vi "GetIntegrationMetaData.vi"(8 "error in":errorcluster, 11 "Datawarehouse in":refnum<class "Datawarehouse.lvclass">) -> (0 "error out":errorcluster, 2 "IntegrationMetaData":string, 3 "Datawarehouse out":refnum<class "Datawarehouse.lvclass">)   [LabVIEW 2021, in "ProligentXMLGenerator.lvlib" / "Datawarehouse.lvclass"]
doc: "The information contained in this attribute is saved in the data warehouse as is. It can\nbe used by the integrator to add some meta data that will help him later to troubleshoot his\nintegration. This meta data is stored in the F_INTEGRATION_METADATA column of the T_FACT_DELIVERY_SOURCE\ntable.\n\nThis value is limited to 2000 charactesrs and must no be empty."
uses:
  Datawarehouse.lvclass
  Datawarehouse.lvclass/Datawarehouse.ctl
  Base/NonEmptyString_2000/NonEmptyString_2000.lvclass
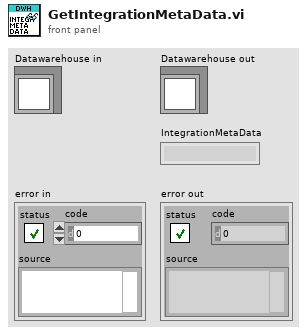
[diagram p1: front panel]
types:
  T1 = typedef "ProligentXMLGenerator.lvlib/Datawarehouse.lvclass/Data.ctl" = cluster{"DestinationFolder":path, "BaseFileName":string, "Document":refnum<k20>, "Defects":refnum<class "Defect.lvclass">[], "TopProcessRuns":refnum<class "ProcessRun.lvclass">[], "ProductUnits":refnum<class "ProductUnit.lvclass">[], "GenerationTime":refnum<class "DateTime.lvclass">, "DataSourceFingerprint":refnum<class "NonEmptyString_448.lvclass">, "IntegrationMetaData":refnum<class "NonEmptyString_2000.lvclass">, "TimeZoneInfoId":string}
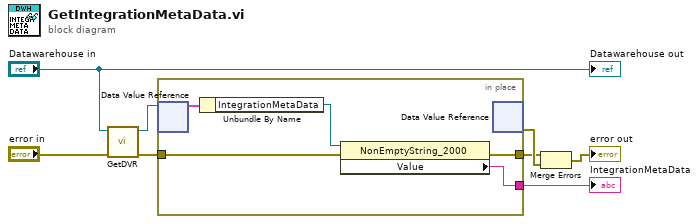
[diagram p0: block diagram]
diagram:
  n1 = call "GetDVR.vi"("error in"="error in", "Datawarehouse"="Datawarehouse in") -> ("error out"=w5:errorcluster, "DVRReference"=w1:refnum<data-value>)  [unwired: 8 in]
  n2 = in-place "In Place Element Structure" {
    in-place-border: w5 -> [w9]
    in-place-border: [w12] -> w4
    in-place-border: [w11] -> w2
    n3 = in-place-dvr #1(w1) -> (w13:T1)  [unwired: 1 out]
    n4 = Unbundle By Name(w13) -> ("IntegrationMetaData"=w10:refnum<class "NonEmptyString_2000.lvclass">)
    n5 = property on="Property Node" class="NonEmptyString_2000"(reference=w10, error in=w9) -> (error out=w12:errorcluster, "Value"=w11:string)  [unwired: 1 out]
    n6 = in-place-dvr #1() -> (w8:errorcluster)  [unwired: 1 in, 1 out]
  }
  "IntegrationMetaData" <- w2
  n7 = Merge Errors(w4, w8) -> (→"error out":errorcluster)
  "Datawarehouse out" <- "Datawarehouse in"
